vi "read raw file info sample rate.vi"(10 "dest":u32, 11 "file":string) -> (2 "dest out":u32, 3 "function return":i32)   [LabVIEW 2019, in "apdm.lvlib"]
doc: "APDM_EXPORT int apdm_read_raw_file_info_sample_rate(const char *file, uint32_t *dest);"
uses:
  apdm.lvlib
  Lee Lab/CP FES Walking 2018/Code/Working/LabVIEW/apdm.dll
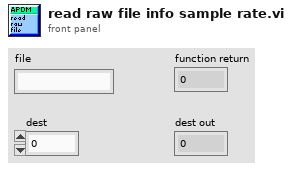
[diagram p1: front panel]
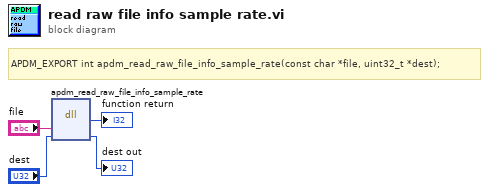
[diagram p0: block diagram]
diagram:
  # "APDM_EXPORT int apdm_read_raw_file_info_sample_rate(const char *file, uint32_t *dest);"
  n1 = dll-call lib="C:/Users/jfalesi/Dropbox/Lee Lab/CP FES Walking 2018/Code/Working/LabVIEW/apdm.*" fn="apdm_read_raw_file_info_sample_rate"("file"="file", "dest"="dest") -> (→"function return":i32, "dest"=→"dest out":u32)  [unwired: 4 in, 2 out]
